vi "Save Waveform List to File.vi"(8 "error in (no error)":errorcluster, 11 "Original Waveforms":waveform(dbl)[](array[waveform])) -> (0 "error out":errorcluster)   [LabVIEW 2021]
uses:
  <vilib>/ErrorRing/Error Ring.xnode
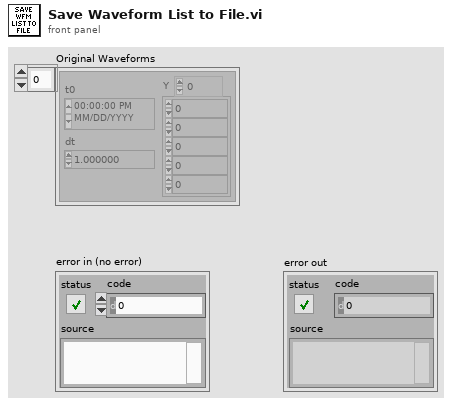
[diagram p1: front panel]
types:
  T1 = enum16{"open", "open or create", "create or replace", "create", "open (read-only)"}
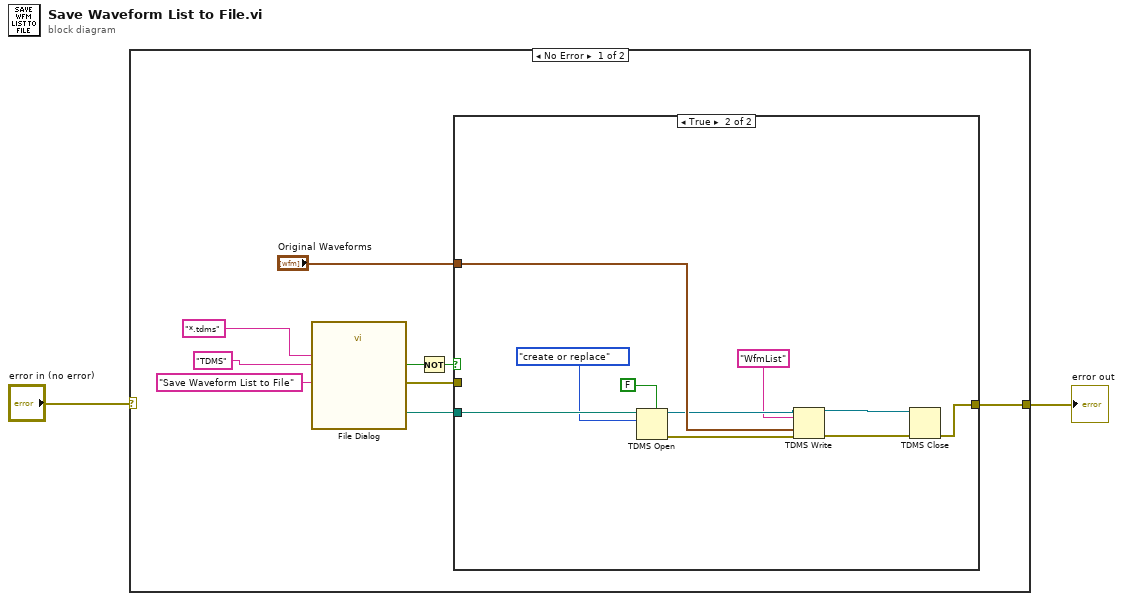
[diagram p0: block diagram]
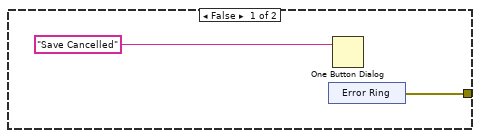
[diagram p2: hidden frame]
diagram:
  n1 = case shown="No Error" "error in (no error)" {
    selector: "error in (no error)" -> [_ w25]
    tunnel: [w3 w25] -> w2
    frame No Error {
      n2 = call "File Dialog"("prompt"="Save Waveform List to File", "pattern (all files)"="*.tdms" ("prompt"), "pattern label"="TDMS" ("prompt")) -> ("selected path"=w8:path, "cancelled"=w7:bool, "error out"=w5:errorcluster)  [unwired: 9 in, 1 out]
      n3 = Not(x=w7) -> (.not. x?=w6:bool)
      n4 = case shown="True" w6 {
        tunnel: w8 -> [_ w24]
        tunnel: w5 -> [_ _]
        tunnel: "Original Waveforms" -> [_ w21]
        tunnel: [w12 w16] -> w3
        frame False {
          n5 = xnode "Error Ring"() -> ("error out"=w12:errorcluster)
          n6 = One Button Dialog(message="Save Cancelled") -> ()  [unwired: 1 in, 1 out]
        }
        frame True {
          n7 = TDMS Open(5:FALSE ("create index file? (T)"), 10:T1."create or replace" ("operation (0:open)"), 11:w24) -> (0:w19:errorcluster, 3:w20:refnum<k34>)  [unwired: 4 in]
          n8 = TDMS Write(0:w20, 5:"WfmList", 9:w21, 11:w19) -> (4:w17:refnum<k34>, 15:w18:errorcluster)  [unwired: 2 in, 2 out]
          n9 = TDMS Close(8:w18, 11:w17) -> (0:w16:errorcluster)  [unwired: 1 out]
        }
      }
    }
    frame Error {
    }
  }
  "error out" <- w2
